vi "MB Globals.vi"() -> ()   [LabVIEW 2023, in "Voegtlin_NI_SMART_Modbus_Drivers.lvlib"]
uses:
  Voegtlin_NI_SMART_Modbus_Drivers.lvlib
panel:
  in  "Allow Access List":string[](array[string])=["*"]
  in  "Max Connections Non-priority":i32=10
  in  "Max Connections Priority":i32=10
  in  "Priority Connection Pool Addresses":string[](array[string])
  in  "Denied Access List":string[](array[string])
  in  "Ethernet Demon Running":bool=TRUE
  in  "Serial Demon Running":bool=TRUE
  in  "Server Loop Rate":u32=200
  in  "Slave Address":u8=1
  in  "Exception Status":u8
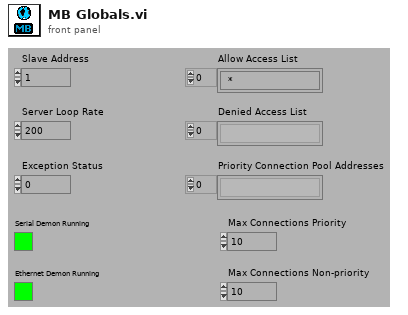
[diagram p1: front panel]
diagram:
